vi "TimerCounter.vi"(4 "NoTriggerState?":bool, 6 "LoopRate(ms)":u16=100, 8 "CounterTime(s)":dbl=0.5, 10 "TriggerStatus":bool) -> (1 "CountersN":u16, 2 "ResultOutput":bool)   [LabVIEW 2019, in "sbRIO9623.lvlib"]
uses:
  sbRIO9623.lvlib
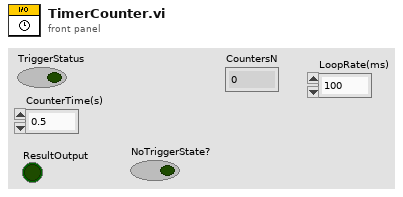
[diagram p1: front panel]
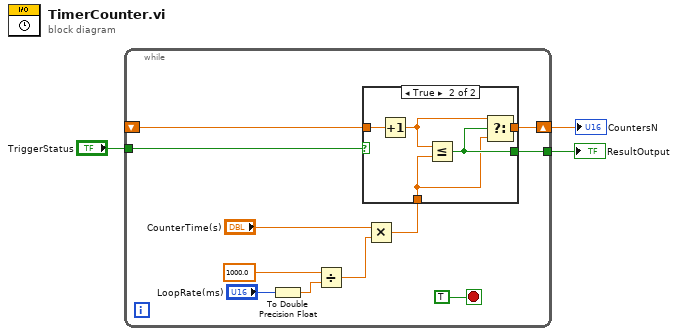
[diagram p0: block diagram]
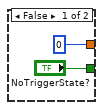
[diagram p2: hidden frame]
diagram:
  n1 = while {
    tunnel: "TriggerStatus" -> [w14]
    tunnel: [w13] -> w2
    shift-right: [w11] -> w1
    shift-left: _ -> [w10]
    stop <- TRUE stop-if-true
    n2 = To Double Precision Float(number="LoopRate(ms)") -> (double precision float=w7:dbl)
    n3 = Divide(x=1000.0, y=w7) -> (x/y=w5:dbl)
    n4 = Multiply(x="CounterTime(s)", y=w5) -> (x*y=w4:dbl)
    n5 = case shown="True" w14 {
      tunnel: [u16 0 w18] -> w11
      tunnel: w10 -> [_ w21]
      tunnel: ["NoTriggerState?" w20] -> w13
      tunnel: w4 -> [_ w17]
      frame False {
      }
      frame True {
        n6 = Increment(x=w21) -> (x+1=w19:dbl)
        n7 = Less Or Equal?(x=w19, y=w17) -> (x <= y?=w20:bool)
        n8 = Select(t=w19, s=w20, f=w17) -> (s? t:f=w18:dbl)
      }
    }
  }
  "ResultOutput" <- w2
  "CountersN" <- w1
